vi "Teleop.vi"(10 "Match Info":T1={"Autonomous Elapsed Seconds"=0.0, "TeleOp Elapsed Seconds"=0.0, "Disabled Elapsed Seconds"=0.0, "Visited Autonomous"=FALSE, "Visited TeleOp"=FALSE, "Visited Disabled"=FALSE, "Autonomous Settings"={"Autonomous Style"=enum."Independent", "VI Refnum"=refnum}}, 11 "Call Context":T2) -> ()   [LabVIEW 2012]
doc: "This VI is called for each TeleOp packet received from the DS where the robot is not disabled. It is often used to read from the joysticks and update I/O or to update setpoints for timed control loops. It should complete and return within 20 milliseconds or it may miss DS packets."
uses:
  <vilib>/Rock Robotics/WPI/DriverStation/WPI_DriverStationDerivedRobotMode.ctl
  <vilib>/Rock Robotics/WPI/DriverStation/WPI_DriverStationMatch Info.ctl
  Robot Global Data.vi
  <vilib>/addons/control/pid/pid.llb/PID Output Rate Limiter (DBL).vi
  <vilib>/Rock Robotics/WPI/Joystick/WPI_JoystickGetSetRefNum.vi
  <vilib>/Rock Robotics/WPI/RobotDrive/WPI_RobotDriveGetSetRefNum.vi
  <vilib>/addons/control/pid/NI_PID_pid.lvlib
panel:
  in  "Boolean":bool
  out "Numeric 1":dbl(slide) scale=0.0..100.0
  out "Boolean 2":bool
  out "Boolean 1":bool
  # "True: Curve\nFalse: Raw"
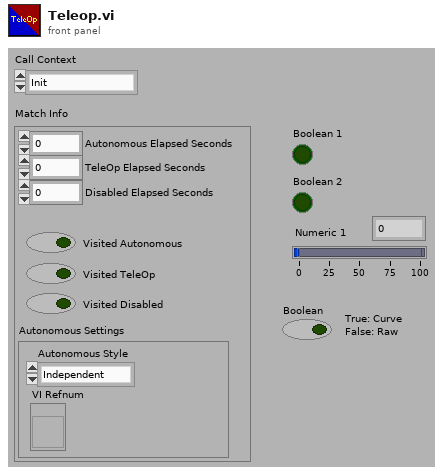
[diagram p1: front panel]
types:
  T1 = typedef "WPI_DriverStationMatch Info.ctl" = cluster{"Autonomous Elapsed Seconds":dbl, "TeleOp Elapsed Seconds":dbl, "Disabled Elapsed Seconds":dbl, "Visited Autonomous":bool, "Visited TeleOp":bool, "Visited Disabled":bool, "Autonomous Settings":cluster{"Autonomous Style":enum16{"Iterative", "Independent"}, "VI Refnum":refnum<vi>}}
  T2 = typedef "WPI_DriverStationDerivedRobotMode.ctl" = enum16{"Init", "Execute", "Stop"}
  T3 = typedef "WPI_RobotDriveDevRef.ctl" = cluster{"DevStatus":errorcluster, "Motors[]":T4[], "Square Inputs":bool, "Max Output":dbl, "Isochronous":bool}
  T4 = typedef "WPI_MotorControlDeviceRef.ctl" = cluster{"DeviceStatus":errorcluster, "Type":enum16{"PWM", "CAN"}, "PWM":cluster{"Digital Module":T5, "PWM Channel":T6, "DeadBand":T7}, "CAN":cluster{"Device Number":u8, "Control Mode":T8, "Semaphore":T9, "Max Vout":dbl}, "Invert":bool, "TransformRef":T10, "InvTransformRef":T10}
  T5 = typedef "FPGA_TypedefDigitalModule.ctl" = enum16{"Digital Module 1", "Digital Module 2"}
  T6 = typedef "FPGA_DIOPWMChannel.ctl" = enum8{"PWM 1", "PWM 2", "PWM 3", "PWM 4", "PWM 5", "PWM 6", "PWM 7", "PWM 8", "PWM 9", "PWM 10", "Invalid"}
  T7 = typedef "WPI_PWMDeadband.ctl" = cluster{"Name":string, "maxPositivePwm":i32, "minPositivePwm":i32, "centerPwm":i32, "maxNegativePwm":i32, "minNegativePwm":i32, "angularRange":u16}
  T8 = typedef "WPI_CANJaguar_ControlMode.ctl" = enum8{"Percent VBus", "Current", "Speed", "Position", "Voltage"}
  T9 = typedef "Semaphore RefNum" = refnum<k1>
  T10 = typedef "WPI_PWMTransform_ConPane.ctl" = refnum<vi>
  T11 = typedef "WPI_JoystickDevRef.ctl" = cluster{"Device":T12}
  T12 = typedef "WPI_JoystickDeviceEnum.ctl" = enum16{"USB 1", "USB 2", "USB 3", "USB 4", "Kinect 1", "Kinect 2"}
  T13 = cluster{"axis 1 (x)":dbl, "axis 2 (y)":dbl, "axis 3 (throttle)":dbl, "axis 4":dbl, "axis 5":dbl, "axis 6":dbl}
  T14 = typedef "WPI_JoystickButtonState.ctl" = cluster{"Button 1":bool, "Button 2":bool, "Button 3":bool, "Button 4":bool, "Button 5":bool, "Button 6":bool, "Button 7":bool, "Button 8":bool, "Button 9":bool, "Button 10":bool, "Button 11":bool, "Button 12":bool}
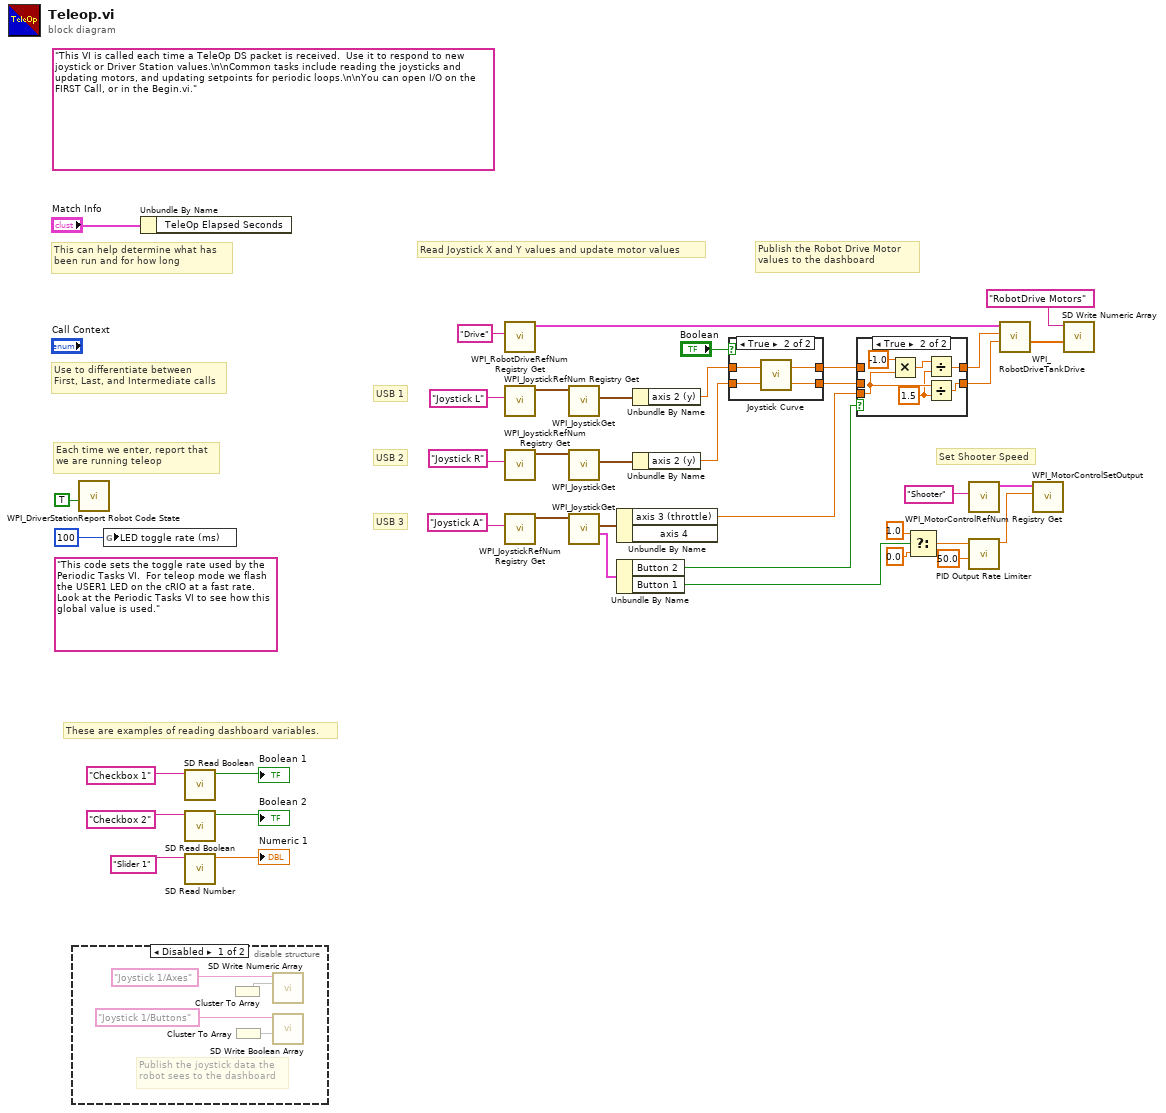
[diagram p0: block diagram]
diagram:
  (unwired) "This code sets the toggle rate used by the Periodic Tasks VI.  For teleop mode we flash the USER1 LED on the cRIO at a fast rate.  Look at the Periodic Tasks VI to see how this global value is used."
  (unwired) "This VI is called each time a TeleOp DS packet is received.  Use it to respond to new joystick or Driver Station values.\n\nCommon tasks include reading the joysticks and updating motors, and updating setpoints for periodic loops.\n\nYou can open I/O on the FIRST Call, or in the Begin.vi."
  # "USB 3"
  # "Set Shooter Speed"
  # "USB 2"
  # "USB 1"
  # "These are examples of reading dashboard variables."
  # "Publish the Robot Drive Motor\nvalues to the dashboard"
  # "Each time we enter, report that\nwe are running teleop"
  # "Use to differentiate between\nFirst, Last, and Intermediate calls"
  # "This can help determine what has\nbeen run and for how long"
  # "Read Joystick X and Y values and update motor values"
  n1 = disable-structure shown="Disabled" {
    frame Disabled {
      # "Publish the joystick data the\nrobot sees to the dashboard"
      n2 = Cluster To Array() -> (array=w42:void[])  [unwired: 1 in]
      n3 = Cluster To Array() -> (array=w44:void[])  [unwired: 1 in]
      n4 = call <vilib>:"SD Write Numeric Array.vi"("Numeric Array"=w42, "Name"="Joystick 1/Axes") -> ()  [unwired: 8 in, 2 out]
      n5 = call <vilib>:"SD Write Boolean Array.vi"("Boolean Array"=w44, "Name"="Joystick 1/Buttons") -> ()  [unwired: 8 in, 2 out]
    }
    frame Enabled {
    }
  }
  n6 = call <vilib>:"WPI_DriverStationReport Robot Code State.vi"("TeleOp"=TRUE ("Autonomous")) -> ()  [unwired: 10 in, 1 out]
  n7 = global write "Robot Global Data.vi" "LED toggle rate (ms)"(u32 100 ("LED ms toggle rate")) -> ()
  n8 = Unbundle By Name("Match Info") -> ()  [unwired: 1 out]
  n9 = call <vilib>:"SD Read Boolean.vi"("Name"="Checkbox 1" ("refnum name")) -> ("Boolean"=→"Boolean 1":bool)  [unwired: 8 in, 2 out]
  n10 = call <vilib>:"SD Read Boolean.vi"("Name"="Checkbox 2" ("refnum name")) -> ("Boolean"=→"Boolean 2":bool)  [unwired: 8 in, 2 out]
  n11 = call <vilib>:"SD Read Number.vi"("Name"="Slider 1" ("refnum name")) -> ("Numeric"=→"Numeric 1":dbl)  [unwired: 8 in, 2 out]
  n12 = call <vilib>:"WPI_RobotDriveRefNum Registry Get.vi"("refnum name"="Drive") -> ("RobotDriveDevRef"=w13:T3)  [unwired: 1 in, 9 out]
  n13 = call <vilib>:"WPI_JoystickRefNum Registry Get.vi"("refnum name"="Joystick L") -> ("JoystickDevRef"=w37:T11)  [unwired: 1 in, 9 out]
  n14 = call <vilib>:"WPI_JoystickRefNum Registry Get.vi"("refnum name"="Joystick R") -> ("JoystickDevRef"=w24:T11)  [unwired: 1 in, 9 out]
  n15 = call <vilib>:"WPI_JoystickRefNum Registry Get.vi"("refnum name"="Joystick A") -> ("JoystickDevRef"=w19:T11)  [unwired: 1 in, 9 out]
  n16 = call <vilib>:"WPI_JoystickGet.vi"("JoystickDevRef"=w37) -> ("Axes"=w34:T13)  [unwired: 1 in, 5 out]
  n17 = call <vilib>:"WPI_JoystickGet.vi"("JoystickDevRef"=w24) -> ("Axes"=w23:T13)  [unwired: 1 in, 5 out]
  n18 = call <vilib>:"WPI_JoystickGet.vi"("JoystickDevRef"=w19) -> ("Buttons"=w14:T14, "Axes"=w18:T13)  [unwired: 1 in, 4 out]
  n19 = Unbundle By Name(w18) -> ("axis 3 (throttle)"=w7:dbl)  [unwired: 1 out]
  n20 = Unbundle By Name(w14) -> ("Button 2"=w8:bool, "Button 1"=w6:bool)
  n21 = Unbundle By Name(w34) -> ("axis 2 (y)"=w15:dbl)
  n22 = Unbundle By Name(w23) -> ("axis 2 (y)"=w16:dbl)
  n23 = case shown="True" "Boolean" {
    tunnel: w16 -> [w46 w50]
    tunnel: [w46 w49] -> w10
    tunnel: w15 -> [w45 w48]
    tunnel: [w45 w47] -> w11
    frame False {
    }
    frame True {
      n24 = call "Joystick Curve.vi"("Right Axis Value"=w50, "Left Axis Value"=w48) -> ("Modified Right Axis Value"=w49:dbl, "Modified Left Axis Value"=w47:dbl)
    }
  }
  n25 = case shown="True" w8 {
    tunnel: [w52 w53] -> w12
    tunnel: w11 -> [w52 _]
    tunnel: [w51 w54] -> w9
    tunnel: w10 -> [w51 _]
    tunnel: w7 -> [_ w56]
    frame False {
    }
    frame True {
      w55 = 1.5 ("y")
      n26 = Multiply(x=-1.0, y=w56) -> (x*y=w57:dbl)
      n27 = Divide(x=w57, y=w55) -> (x/y=w53:dbl)
      n28 = Divide(x=w56, y=w55) -> (x/y=w54:dbl)
    }
  }
  n29 = Select(t=1.0, s=w6, f=0.0) -> (s? t:f=w3:dbl)
  n30 = call <vilib>:"WPI_MotorControlRefNum Registry Get.vi"("refnum name"="Shooter") -> ("MotorControlDevRef"=w21:T4)  [unwired: 9 in, 1 out]
  n31 = call-poly <vilib>:"PID Output Rate Limiter.vi"("output rate (EGU/min)"=50.0, "input (controller output)"=w3) -> ("output"=w2:dbl)  [unwired: 6 in, 1 out]
  n32 = call <vilib>:"WPI_RobotDriveTankDrive.vi"("Right axis value"=w9, "Left axis value"=w12, "RobotDriveDevRef"=w13) -> ("Motor Values"=w32:dbl[])  [unwired: 6 in, 2 out]
  n33 = call <vilib>:"WPI_MotorControlSetOutput.vi"("Output"=w2, "MotorControlDevRef"=w21) -> ()  [unwired: 7 in, 3 out]
  n34 = call <vilib>:"SD Write Numeric Array.vi"("Numeric Array"=w32, "Name"="RobotDrive Motors") -> ()  [unwired: 8 in, 2 out]
